vi "Normaliz3.1.vi"(10 "data info template":T1={"data path"="", "ADCintercadr_s"=1.0, "data info"={"use or not *.info.txt?"=0, "probe name"="NaN", "signal type"="NaN", "Unit"="NaN", "variable"="NaN", "attenuation factor"=1.0, "amplification factor"=1.0, "extracoef#1"=1.0, "extracoef#2"=1.0, "U cascade, kV"="NaN", "probe area, cm2"=1.0, "plasma, a.m.u."=1.0}, "channel_name"="", "channels_in_file"=0}, 11 "Array in":waveform(dbl)[](array[waveform])) -> (3 "Array out":waveform(dbl)[](array[waveform]))   [LabVIEW 2014]
uses:
  <vilib>/measure/mascope.llb/Amplitude and Levels 1 chan.vi
  <vilib>/measure/NI_MAPro.lvlib
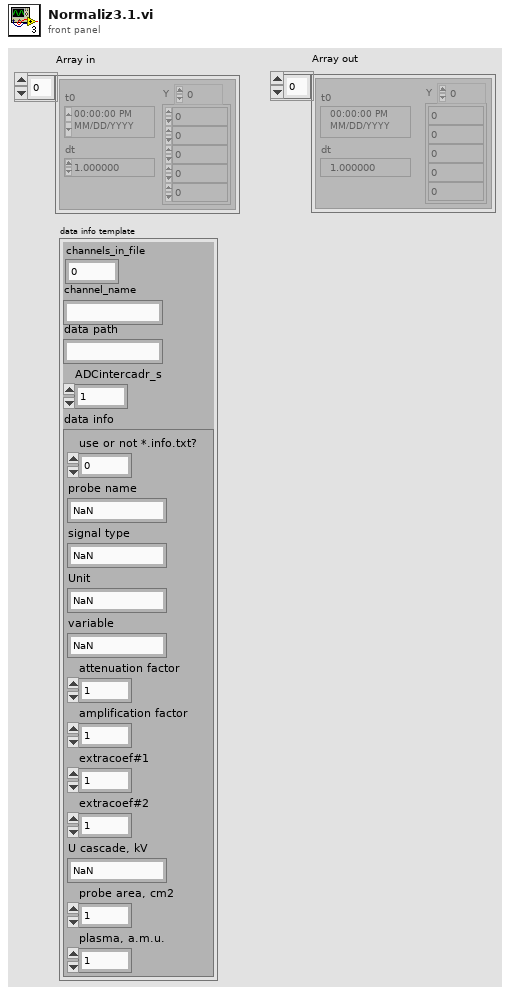
[diagram p1: front panel]
types:
  T1 = cluster{"data path":string, "ADCintercadr_s":dbl, "data info":cluster{"use or not *.info.txt?":i16, "probe name":string, "signal type":string, "Unit":string, "variable":string, "attenuation factor":dbl, "amplification factor":dbl, "extracoef#1":dbl, "extracoef#2":dbl, "U cascade, kV":string, "probe area, cm2":dbl, "plasma, a.m.u.":dbl}, "channel_name":string, "channels_in_file":i32}
  T2 = cluster{"method":enum32{"histogram", "peak", "auto select"}, "histogram size":i32, "histogram method":enum16{"mode"}, "reserved":dbl}
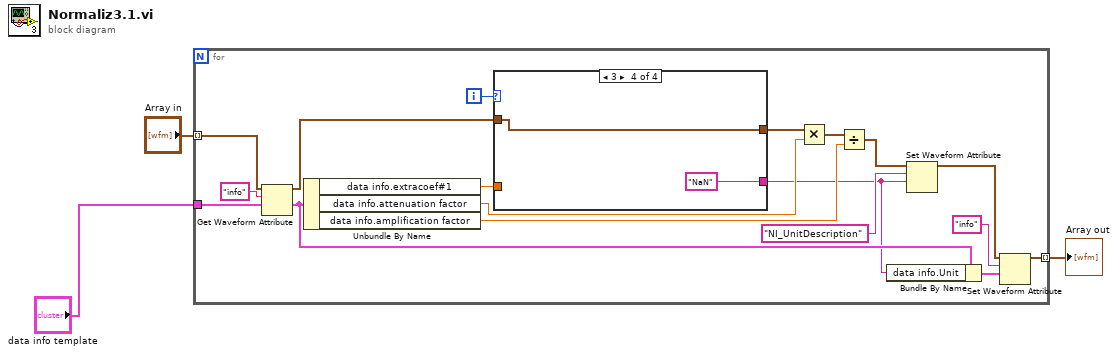
[diagram p0: block diagram]
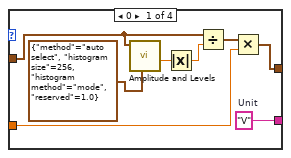
[diagram p2: hidden frame]
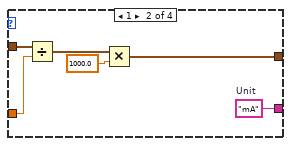
[diagram p3: hidden frame]
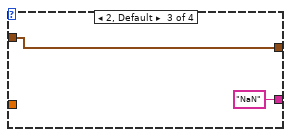
[diagram p4: hidden frame]
diagram:
  n1 = for {
    tunnel: [w6] -> w3 mode=indexing
    tunnel: "Array in" -> [w5] mode=indexing
    tunnel: "data info template" -> [w4]
    i -> [w7]
    n2 = Get Waveform Attribute(5:w4, 6:"info" ("name"), 7:w5) -> (1:w10:T1, 3:w21:waveform(dbl))  [unwired: 1 in, 2 out]
    n3 = Unbundle By Name(w10) -> ("data info.extracoef#1"=w13:dbl, "data info.attenuation factor"=w15:dbl, "data info.amplification factor"=w16:dbl)
    n4 = case shown="3" w7 {
      tunnel: w21 -> [w28 w34 w37 w39]
      tunnel: [w23 w30 w37 w39] -> w19
      tunnel: [w25 w35 "NaN" ("Unit") "NaN" ("Unit")] -> w9
      tunnel: w13 -> [w22 w33 _ _]
      frame 0 {
        w25 = "V"  # Unit
        n5 = call-poly <vilib>:"Amplitude and Levels.vi"("state settings"=T2 {"method"=enum."auto select", "histogram size"=256, "histogram method"=enum."mode", "reserved"=1.0}, "signal in"=w28) -> ("low state level"=w27:dbl)  [unwired: 6 in, 3 out]
        n6 = Absolute Value(x=w27) -> (abs(x)=w29:dbl)
        n7 = Divide(x=w28, y=w29) -> (x/y=w24:waveform(dbl))
        n8 = Multiply(x=w24, y=w22) -> (x*y=w23:waveform(dbl))
      }
      frame 1 {
        w35 = "mA"  # Unit
        n9 = Divide(x=w34, y=w33) -> (x/y=w32:waveform(dbl))
        n10 = Multiply(x=w32, y=1000.0) -> (x*y=w30:waveform(dbl))
      }
      frame 2, Default {
      }
      frame 3 {
      }
    }
    n11 = Multiply(x=w19, y=w15) -> (x*y=w17:waveform(dbl))
    n12 = Divide(x=w17, y=w16) -> (x/y=w14:waveform(dbl))
    n13 = Bundle By Name(cluster=w10, "data info.Unit"=w9) -> (w8:T1)
    n14 = Set Waveform Attribute(5:w9, 6:"NI_UnitDescription" ("name"), 7:w14) -> (3:w12:waveform(dbl))  [unwired: 1 in, 2 out]
    n15 = Set Waveform Attribute(5:w8, 6:"info" ("name"), 7:w12) -> (3:w6:waveform(dbl))  [unwired: 1 in, 2 out]
  }
  "Array out" <- w3
